vi "gvbooleschRT.vi"() -> ()   [LabVIEW 2017, in "Licor-Steuerung.lvlib"]
uses:
  Licor-Steuerung.lvlib
panel:
  in  "global stop RT":bool
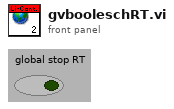
[diagram p1: front panel]
diagram:
